vi "1C Wind Calculations.vi"(7 "Boat Heading":T3 format="%05.1f", 8 "Boat Velocity":T2, 9 "Absolute Wind":T2, 10 "Add Randomness\nTo Wind Measurement":bool) -> (1 "Apparent Wind Speed":T4, 2 "Apparent Wind\nDirection":T5, 3 "Apparent Wind":T1)   [LabVIEW 2011]
doc: "Given absolute wind, boat velocity and heading, produces apparent wind data. Also places this data on the global."
uses:
  2-Think/2 Typedefs/Velocity.ctl
  2-Think/2 Typedefs/apparent wind direction.ctl
  2-Think/2 Typedefs/apparent wind speed.ctl
  2-Think/2 Typedefs/heading.ctl
  2-Think/2 Typedefs/apparent wind.ctl
  2-Think/2 Globals/2 Global.vi
panel:
  out "Apparent Wind\nin global rotation frame":T2
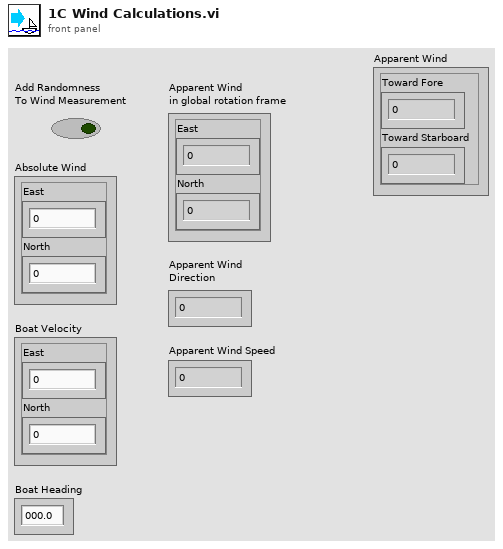
[diagram p1: front panel]
types:
  T1 = typedef "apparent wind.ctl" = cluster{"Toward Fore":dbl, "Toward Starboard":dbl}
  T2 = typedef "Velocity.ctl" = cluster{"East":dbl, "North":dbl}
  T3 = typedef "heading.ctl" = dbl
  T4 = typedef "apparent wind speed.ctl" = dbl
  T5 = typedef "apparent wind direction.ctl" = dbl
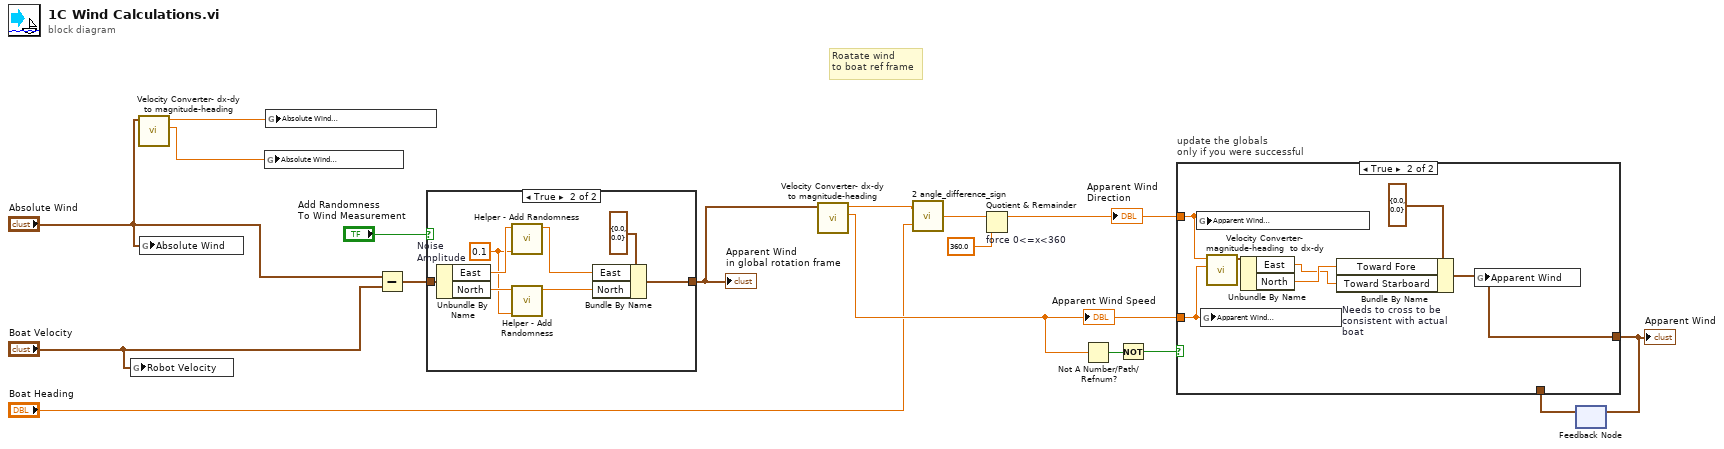
[diagram p0: block diagram]
diagram:
  # "Roatate wind\nto boat ref frame"
  n1 = global write "2 Global.vi" "Robot Velocity"("Boat Velocity") -> ()
  n2 = call "Velocity Converter- dx-dy to magnitude-heading.vi"("Vector In"="Absolute Wind") -> ("Magnitude Out"=w16:dbl, "Heading Out"=w17:T3)  [unwired: 9 in]
  n3 = global write "2 Global.vi" "Absolute Wind"("Absolute Wind") -> ()
  n4 = global write "2 Global.vi" "Absolute Wind\nSpeed"(w16) -> ()
  n5 = global write "2 Global.vi" "Absolute Wind\nDirection (º)"(w17) -> ()
  n6 = Subtract(x="Absolute Wind", y="Boat Velocity") -> (x-y=w11:T2)
  n7 = case shown="True" "Add Randomness\nTo Wind Measurement" {
    tunnel: [w18 w26] -> w8
    tunnel: w11 -> [w18 w25]
    frame False {
    }
    frame True {
      w20 = 0.1  # Noise Amplitude
      n8 = Unbundle By Name(w25) -> ("East"=w24:dbl, "North"=w23:dbl)
      n9 = call "Helper - Add Randomness.vi"("Amplitude\n(default 1)"=w20, "Numeric in"=w24) -> ("Numeric out"=w21:dbl)  [unwired: 9 in]
      n10 = call "Helper - Add Randomness.vi"("Amplitude\n(default 1)"=w20, "Numeric in"=w23) -> ("Numeric out"=w22:dbl)  [unwired: 9 in]
      n11 = Bundle By Name(cluster=T2 {"East"=0.0, "North"=0.0} ("Apparent Wind 2"), "East"=w21, "North"=w22) -> (w26:T2)
    }
  }
  "Apparent Wind\nin global rotation frame" <- w8
  n12 = call "Velocity Converter- dx-dy to magnitude-heading.vi"("Vector In"=w8) -> ("Magnitude Out"=w13:dbl, "Heading Out"=w1:T3)  [unwired: 9 in]
  "Apparent Wind Speed" <- w13
  n13 = call "2 angle_difference_sign.vi"("Angle 2"="Boat Heading", "Angle 1"=w1) -> ("Difference"=w3:dbl)
  n14 = Quotient & Remainder "force 0<=x<360"(x=w3, y=T3 360.0) -> (x-y*floor(x/y)=w12:T3)  [unwired: 1 out]
  "Apparent Wind\nDirection" <- w12
  n15 = Not A Number/Path/Refnum?(number/path/refnum=w13) -> (NaN/Path/Refnum?=w9:bool)
  n16 = Not(x=w9) -> (.not. x?=w10:bool)
  n17 = feedback #1() -> (w4:T1)  [unwired: 1 in]
  n18 = case "update the globals\nonly if you were successful" shown="True" w10 {
    tunnel: w12 -> [_ w34]
    tunnel: w13 -> [_ w33]
    tunnel: [w27 w28] -> w5
    tunnel: w4 -> [w27 _]
    frame False {
    }
    frame True {
      n19 = global write "2 Global.vi" "Apparent Wind\nDirection (º)"(w34) -> ()
      n20 = global write "2 Global.vi" "Apparent Wind\nSpeed"(w33) -> ()
      n21 = call "Velocity Converter- magnitude-heading  to dx-dy.vi"("Magnitude"=w33, "Heading"=w34) -> ("Vector Out"=w32:T2)  [unwired: 9 in]
      n22 = Unbundle By Name(w32) -> ("East"=w29:dbl, "North"=w30:dbl)
      n23 = Bundle By Name "Needs to cross to be consistent with actual boat"(cluster=T1 {"Toward Fore"=0.0, "Toward Starboard"=0.0} ("Apparent Wind"), "Toward Fore"=w30, "Toward Starboard"=w29) -> (w28:T1)
      n24 = global write "2 Global.vi" "Apparent Wind"(w28) -> ()
    }
  }
  "Apparent Wind" <- w5
  n25 = feedback-in #1(w5) -> ()
